vi "FilePathFacade.vi"(0 "Data In":T4, 2 "Display State In":T2, 3 "Container State":T3) -> (6 "Data Out":T4, 7 "Display State Out":T2, 8 "Action":T1)   [LabVIEW 2014, in "FilePathControl.xctl"]
uses:
  <userlib>/CurtinCode/Filexctrl/FilePathControl.xctl
  <userlib>/CurtinCode/Filexctrl/FilePathData.ctl
  <vilib>/_xctls/Container State.ctl
  <userlib>/CurtinCode/Filexctrl/FilePathState.ctl
  <vilib>/_xctls/Action.ctl
  <vilib>/_xctls/XControlSupport.lvlib
panel:
  in  "Path to Data Folder":path
  in  "File Paths":string[](tree)
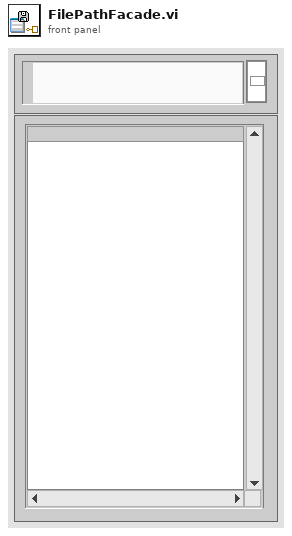
[diagram p1: front panel]
types:
  T1 = typedef "XControlSupport.lvlib/Action.ctl" = cluster{"Data Changed?":bool, "State Changed?":bool, "Action Name":string}
  T2 = typedef "FilePathControl.xctl/FilePathState.ctl" = path
  T3 = typedef "XControlSupport.lvlib/Container State.ctl" = cluster{"Indicator?":bool, "Run Mode?":bool, " Refnum":refnum<vi>}
  T4 = typedef "FilePathControl.xctl/FilePathData.ctl" = path[]
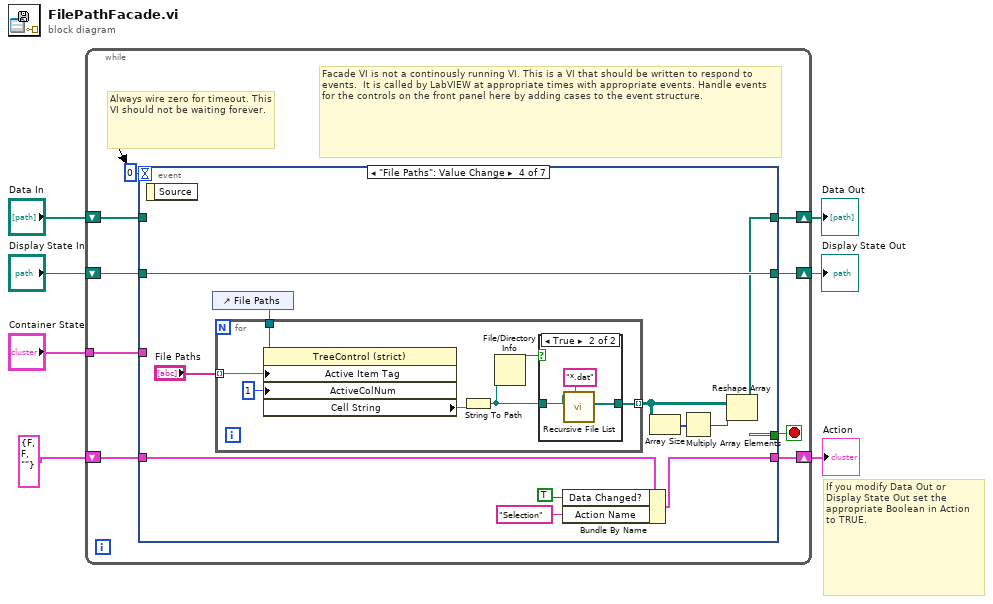
[diagram p0: block diagram]
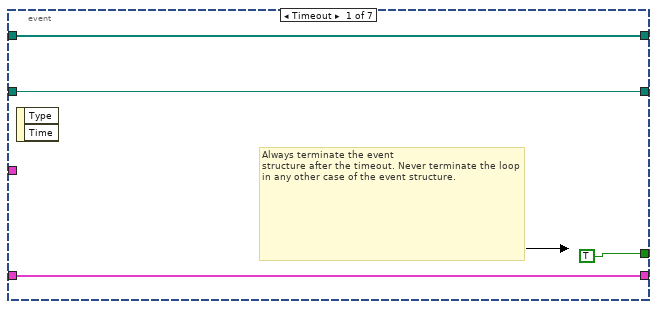
[diagram p2: hidden frame]
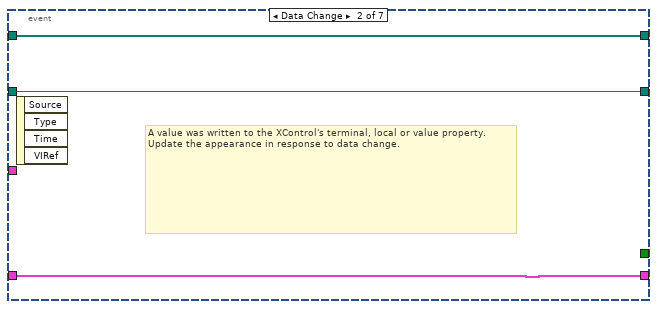
[diagram p3: hidden frame]
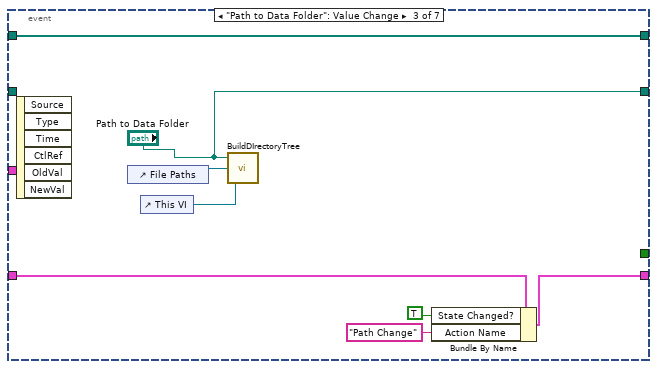
[diagram p4: hidden frame]
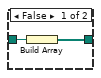
[diagram p5: hidden frame]
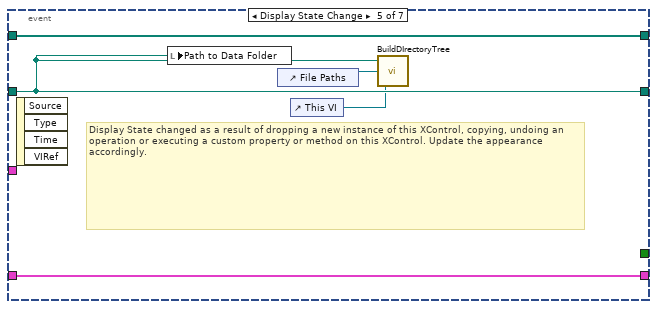
[diagram p6: hidden frame]
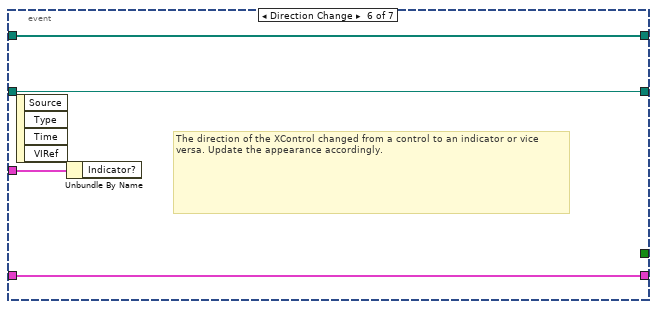
[diagram p7: hidden frame]
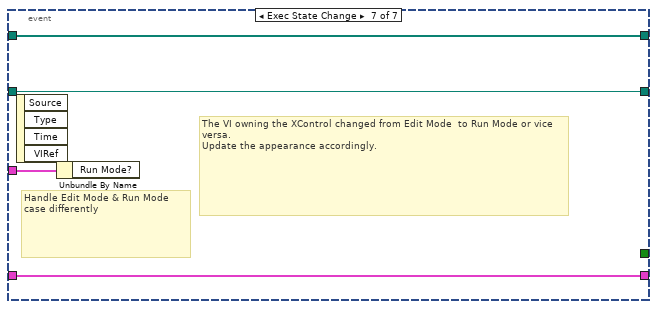
[diagram p8: hidden frame]
diagram:
  # "If you modify Data Out or\nDisplay State Out set the\nappropriate Boolean in Action\nto TRUE."
  n1 = while {
    shift-right: [w15] -> w4
    shift-left: "Display State In" -> [w16]
    tunnel: "Container State" -> [w12]
    shift-right: [w10] -> w7
    shift-left: "Data In" -> [w11]
    shift-right: [w8] -> w2
    shift-left: T1 {"Data Changed?"=FALSE, "State Changed?"=FALSE, "Action Name"=""} ("Action") -> [w9]
    stop <- w14 stop-if-true
    # "Facade VI is not a continously running VI. This is a VI that should be written to respond to events.  It is called by LabVIEW at appropriate times with appropriate events. Handle events for the controls on the front panel here by adding cases to the event structure."
    # "Always wire zero for timeout. This\nVI should not be waiting forever."
    n2 = event shown="[3] \"File Paths\": Value Change" {
      selector: _ -> [_ _ _ _ _ _ _]
      dyn-events: _ -> [_ _ _ _ _ _ _]
      timeout: 0 -> [_ _ _ _ _ _ _]
      tunnel: w16 -> [w18 w22 _ w38 w57 w62 w66]
      tunnel: [w18 w22 "Path to Data Folder" w38 w57 w62 w66] -> w15
      tunnel: [TRUE _ _ _ _ _ _] -> w14
      tunnel: w12 -> [_ _ _ _ _ w63 w67]
      tunnel: w11 -> [w17 w23 w31 _ w59 w61 w65]
      tunnel: [w17 w23 w31 w35 w59 w61 w65] -> w10
      tunnel: [w19 w21 w27 w41 w58 w60 w64] -> w8
      tunnel: w9 -> [w19 w21 w28 w42 w58 w60 w64]
      event Timeout {
        # "Always terminate the event\nstructure after the timeout. Never terminate the loop in any other case of the event structure."
        n3 = event-data() -> ()  [unwired: 1 in, 2 out]
      }
      event Data Change {
        # "A value was written to the XControl's terminal, local or value property.\nUpdate the appearance in response to data change."
        n4 = event-data() -> ()  [unwired: 1 in, 4 out]
      }
      event "Path to Data Folder": Value Change {
        n5 = event-data() -> ()  [unwired: 1 in, 6 out]
        n6 = control-ref of="File Paths"() -> (w29:refnum<vi>)
        n7 = control-ref of="This VI"() -> (w30:refnum<vi>)
        n8 = call <userlib>:"BuildDIrectoryTree.vi"("CallingVI"=w30, "Tree Refnum"=w29, "Folder Path"="Path to Data Folder") -> ()  [unwired: 2 in]
        n9 = Bundle By Name(cluster=w28, "State Changed?"=TRUE ("Data Changed?"), "Action Name"="Path Change") -> (w27:T1)
      }
      event "File Paths": Value Change {
        n10 = event-data() -> ()  [unwired: 1 in, 1 out]
        n11 = control-ref of="File Paths"() -> (w36:refnum<vi>)
        n12 = for {
          tunnel: "File Paths" -> [w49] mode=indexing
          tunnel: [w44] -> w34 mode=indexing
          tunnel: w36 -> [w47]
          n13 = property on="Property Node" class="TreeControl (strict)"(reference=w47, "Active Item Tag"=w49, "ActiveColNum"=1 ("Active Cell:Active Column Number")) -> ("Cell String"=w43:string)  [unwired: 1 in, 2 out]
          n14 = String To Path(string=w43) -> (path=w45:path)
          n15 = File/Directory Info(path=w45) -> (directory=w46:bool)  [unwired: 1 in, 6 out]
          n16 = case shown="True" w46 {
            tunnel: [w50 w52] -> w44
            tunnel: w45 -> [w51 w53]
            frame False {
              n17 = Build Array(w51) -> (w50:path[])
            }
            frame True {
              n18 = call <vilib>:"Recursive File List.vi"("pattern"="*.dat", "Folder Path"=w53) -> ("All Files in Dir"=w52:path[])  [unwired: 5 in, 4 out]
            }
          }
        }
        n19 = Bundle By Name(cluster=w42, "Data Changed?"=TRUE, "Action Name"="Selection") -> (w41:T1)
        n20 = Array Size(array=w34) -> (size(s)=w32:i32[])
        n21 = Multiply Array Elements(1:w32) -> (0:w33:i32)
        n22 = Reshape Array(w34, w33) -> (w35:path[])
      }
      event Display State Change {
        # "Display State changed as a result of dropping a new instance of this XControl, copying, undoing an operation or executing a custom property or method on this XControl. Update the appearance accordingly."
        n23 = event-data() -> ()  [unwired: 1 in, 4 out]
        n24 = local write "Path to Data Folder"(w57) -> ()
        n25 = control-ref of="File Paths"() -> (w56:refnum<vi>)
        n26 = control-ref of="This VI"() -> (w55:refnum<vi>)
        n27 = call <userlib>:"BuildDIrectoryTree.vi"("CallingVI"=w55, "Tree Refnum"=w56, "Folder Path"=w57) -> ()  [unwired: 2 in]
      }
      event Direction Change {
        # "The direction of the XControl changed from a control to an indicator or vice versa. Update the appearance accordingly."
        n28 = event-data() -> ()  [unwired: 1 in, 4 out]
        n29 = Unbundle By Name(w63) -> ()  [unwired: 1 out]
      }
      event Exec State Change {
        # "The VI owning the XControl changed from Edit Mode  to Run Mode or vice versa.\nUpdate the appearance accordingly."
        # "Handle Edit Mode & Run Mode\ncase differently"
        n30 = event-data() -> ()  [unwired: 1 in, 4 out]
        n31 = Unbundle By Name(w67) -> ()  [unwired: 1 out]
      }
    }
  }
  "Display State Out" <- w4
  "Data Out" <- w7
  "Action" <- w2
